vi "HeartBeatLabViewAli.vi"() -> ()   [LabVIEW 2018]
uses:
  <vilib>/Instr/_visa.llb/VISA Configure Serial Port (Instr).vi
panel:
  out "Heart Rate":dbl
  out "Heart Rate":dbl(graph)
  out "Pulse":dbl(graph)
  in  "Serial Port":refnum<visa-resource-name>
  in  "stop":bool
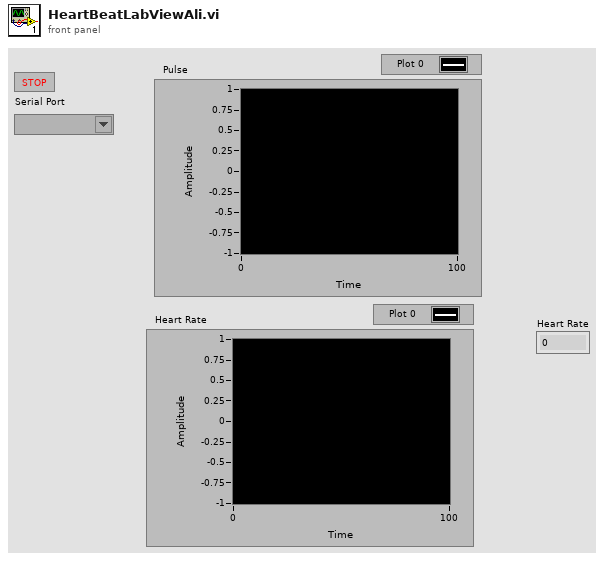
[diagram p1: front panel]
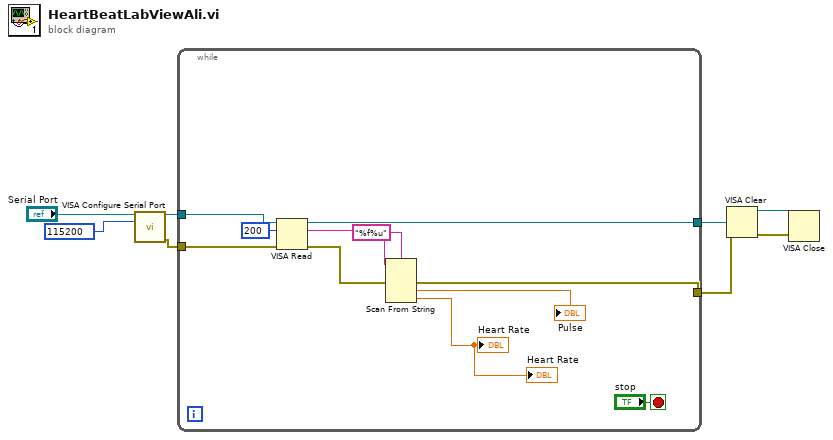
[diagram p0: block diagram]
diagram:
  n1 = call-poly "VISA Configure Serial Port"("VISA resource name"="Serial Port", "baud rate (9600)"=u32 115200) -> ("VISA resource name out"=w8:refnum<visa-resource-name>, "error out"=w7:errorcluster)  [unwired: 12 in]
  n2 = while {
    tunnel: w8 -> [w18]
    tunnel: w7 -> [w17]
    tunnel: [w15] -> w5
    tunnel: [w12] -> w1
    stop <- "stop" stop-if-true
    n3 = VISA Read(VISA resource name=w18, byte count=u32 200, error in (no error)=w17) -> (VISA resource name out=w15:refnum<visa-resource-name>, read buffer=w13:string, error out=w14:errorcluster)  [unwired: 1 out]
    n4 = Scan From String(format string="%f%u", input string=w13, error in=w14) -> (error out=w12:errorcluster, output 1=→"Pulse":dbl, output 2=→"Heart Rate" →"Heart Rate":dbl)  [unwired: 3 in, 2 out]
  }
  n5 = VISA Clear(VISA resource name=w5, error in (no error)=w1) -> (VISA resource name out=w4:refnum<visa-resource-name>, error out=w3:errorcluster)
  n6 = VISA Close(VISA resource name=w4, error in (no error)=w3) -> ()  [unwired: 1 out]
